vi "async worker process.vi"(10 "run flag in":u8 format="%.0b", 11 "module data in":T1={"run state"=enum."sync", "module"=refnum, "module ref"=refnum, "async exec ref"={"command fifo"=refnum, "error fifo"=refnum, "input buffer"=refnum, "output buffer"=refnum, "process buffer"=refnum, "original dvrs"=[]}, "configuration ref"=refnum, "error"={"status"=FALSE, "code"=0, "source"=""}, "previous error code"=0, "input method"={"data table"={"Double"=[], "Single"=[], "I64"=[], "I32"=[], "I16"=[], "I8"=[], "U64"=[], "U32"=[], "U16"=[], "U8"=[], "Boolean"=[], "String"=[], "Array of Double"=[], "Array of Single"=[], "Array of I64"=[], "Array of I32"=[], "Array of I16"=[], "Array of I8"=[], "Array of U64"=[], "Array of U32"=[], "Array of U16"=[], "Array of U8"=[], "Array of Boolean"=[], "Array of String"=[]}, "transfer spec"=[]}, "output method"={"data table"={"Double"=[], "Single"=[], "I64"=[], "I32"=[], "I16"=[], "I8"=[], "U64"=[], "U32"=[], "U16"=[], "U8"=[], "Boolean"=[], "String"=[], "Array of Double"=[], "Array of Single"=[], "Array of I64"=[], "Array of I32"=[], "Array of I16"=[], "Array of I8"=[], "Array of U64"=[], "Array of U32"=[], "Array of U16"=[], "Array of U8"=[], "Array of Boolean"=[], "Array of String"=[]}, "transfer spec"=[]}, "process method parameters"={"data table"={"Double"=[], "Single"=[], "I64"=[], "I32"=[], "I16"=[], "I8"=[], "U64"=[], "U32"=[], "U16"=[], "U8"=[], "Boolean"=[], "String"=[], "Array of Double"=[], "Array of Single"=[], "Array of I64"=[], "Array of I32"=[], "Array of I16"=[], "Array of I8"=[], "Array of U64"=[], "Array of U32"=[], "Array of U16"=[], "Array of U8"=[], "Array of Boolean"=[], "Array of String"=[]}, "transfer spec"=[]}, "process method results"={"data table"={"Double"=[], "Single"=[], "I64"=[], "I32"=[], "I16"=[], "I8"=[], "U64"=[], "U32"=[], "U16"=[], "U8"=[], "Boolean"=[], "String"=[], "Array of Double"=[], "Array of Single"=[], "Array of I64"=[], "Array of I32"=[], "Array of I16"=[], "Array of I8"=[], "Array of U64"=[], "Array of U32"=[], "Array of U16"=[], "Array of U8"=[], "Array of Boolean"=[], "Array of String"=[]}, "transfer spec"=[]}, "fault handling"={"unknown"=[], "trivial"=[], "critical"=[], "recoverable"=[]}, "error report index "=-1}) -> (0 "error out":errorcluster, 2 "run flag out":u8 format="%.0b", 3 "module data out":T1={"run state"=enum."sync", "module"=refnum, "module ref"=refnum, "async exec ref"={"command fifo"=refnum, "error fifo"=refnum, "input buffer"=refnum, "output buffer"=refnum, "process buffer"=refnum, "original dvrs"=[]}, "configuration ref"=refnum, "error"={"status"=FALSE, "code"=0, "source"=""}, "previous error code"=0, "input method"={"data table"={"Double"=[], "Single"=[], "I64"=[], "I32"=[], "I16"=[], "I8"=[], "U64"=[], "U32"=[], "U16"=[], "U8"=[], "Boolean"=[], "String"=[], "Array of Double"=[], "Array of Single"=[], "Array of I64"=[], "Array of I32"=[], "Array of I16"=[], "Array of I8"=[], "Array of U64"=[], "Array of U32"=[], "Array of U16"=[], "Array of U8"=[], "Array of Boolean"=[], "Array of String"=[]}, "transfer spec"=[]}, "output method"={"data table"={"Double"=[], "Single"=[], "I64"=[], "I32"=[], "I16"=[], "I8"=[], "U64"=[], "U32"=[], "U16"=[], "U8"=[], "Boolean"=[], "String"=[], "Array of Double"=[], "Array of Single"=[], "Array of I64"=[], "Array of I32"=[], "Array of I16"=[], "Array of I8"=[], "Array of U64"=[], "Array of U32"=[], "Array of U16"=[], "Array of U8"=[], "Array of Boolean"=[], "Array of String"=[]}, "transfer spec"=[]}, "process method parameters"={"data table"={"Double"=[], "Single"=[], "I64"=[], "I32"=[], "I16"=[], "I8"=[], "U64"=[], "U32"=[], "U16"=[], "U8"=[], "Boolean"=[], "String"=[], "Array of Double"=[], "Array of Single"=[], "Array of I64"=[], "Array of I32"=[], "Array of I16"=[], "Array of I8"=[], "Array of U64"=[], "Array of U32"=[], "Array of U16"=[], "Array of U8"=[], "Array of Boolean"=[], "Array of String"=[]}, "transfer spec"=[]}, "process method results"={"data table"={"Double"=[], "Single"=[], "I64"=[], "I32"=[], "I16"=[], "I8"=[], "U64"=[], "U32"=[], "U16"=[], "U8"=[], "Boolean"=[], "String"=[], "Array of Double"=[], "Array of Single"=[], "Array of I64"=[], "Array of I32"=[], "Array of I16"=[], "Array of I8"=[], "Array of U64"=[], "Array of U32"=[], "Array of U16"=[], "Array of U8"=[], "Array of Boolean"=[], "Array of String"=[]}, "transfer spec"=[]}, "fault handling"={"unknown"=[], "trivial"=[], "critical"=[], "recoverable"=[]}, "error report index "=-1})   [LabVIEW 2013, in "main engine.lvlib"]
doc: "This VI is like a mini data engine for a single TBM. It communicates with the engine that spawned it using a RT FIFO containing a command with DVRs used for data exchange. The command determines what method to run and gets commanded by the engine.\n\nThe engine is therefore still responsible for scheduling the execution of each module, but the engine won't block for data to be returned. An Asynch module can run as fast as an engine, or as slow as is needed to perform the required functionality."
uses:
  main engine/main engine.lvlib
  main engine/full module data.ctl
  <vilib>/NI/Tag Bus Module Framework/runtime/TBM module execution interface.lvclass
  main engine/module run state.ctl
  asynchronous executor reference.ctl
  async message to executor.ctl
  Runtime/async command notification.ctl
  <vilib>/NI/Tag Bus/table/data table.ctl
  Runtime/async error info.ctl
  <vilib>/NI/Tag Bus Module Framework/runtime/error classification.ctl
  <vilib>/NI/Tag Bus Module Framework/module configuration/TBM module configuration.lvclass
  main engine/module method data.ctl
  <vilib>/NI/Tag Bus/table/transfer specification.ctl
  <vilib>/NI/Tag Bus/tag/Data Type.ctl
  main engine/fault handling spec.ctl
  Configuration/Error Actions.ctl
  <vilib>/NI/Tag Bus/table/data table.lvlib
  <vilib>/NI/Tag Bus/tag/tag descriptor.lvclass
  Configuration/Standard Engine Configuration.lvclass
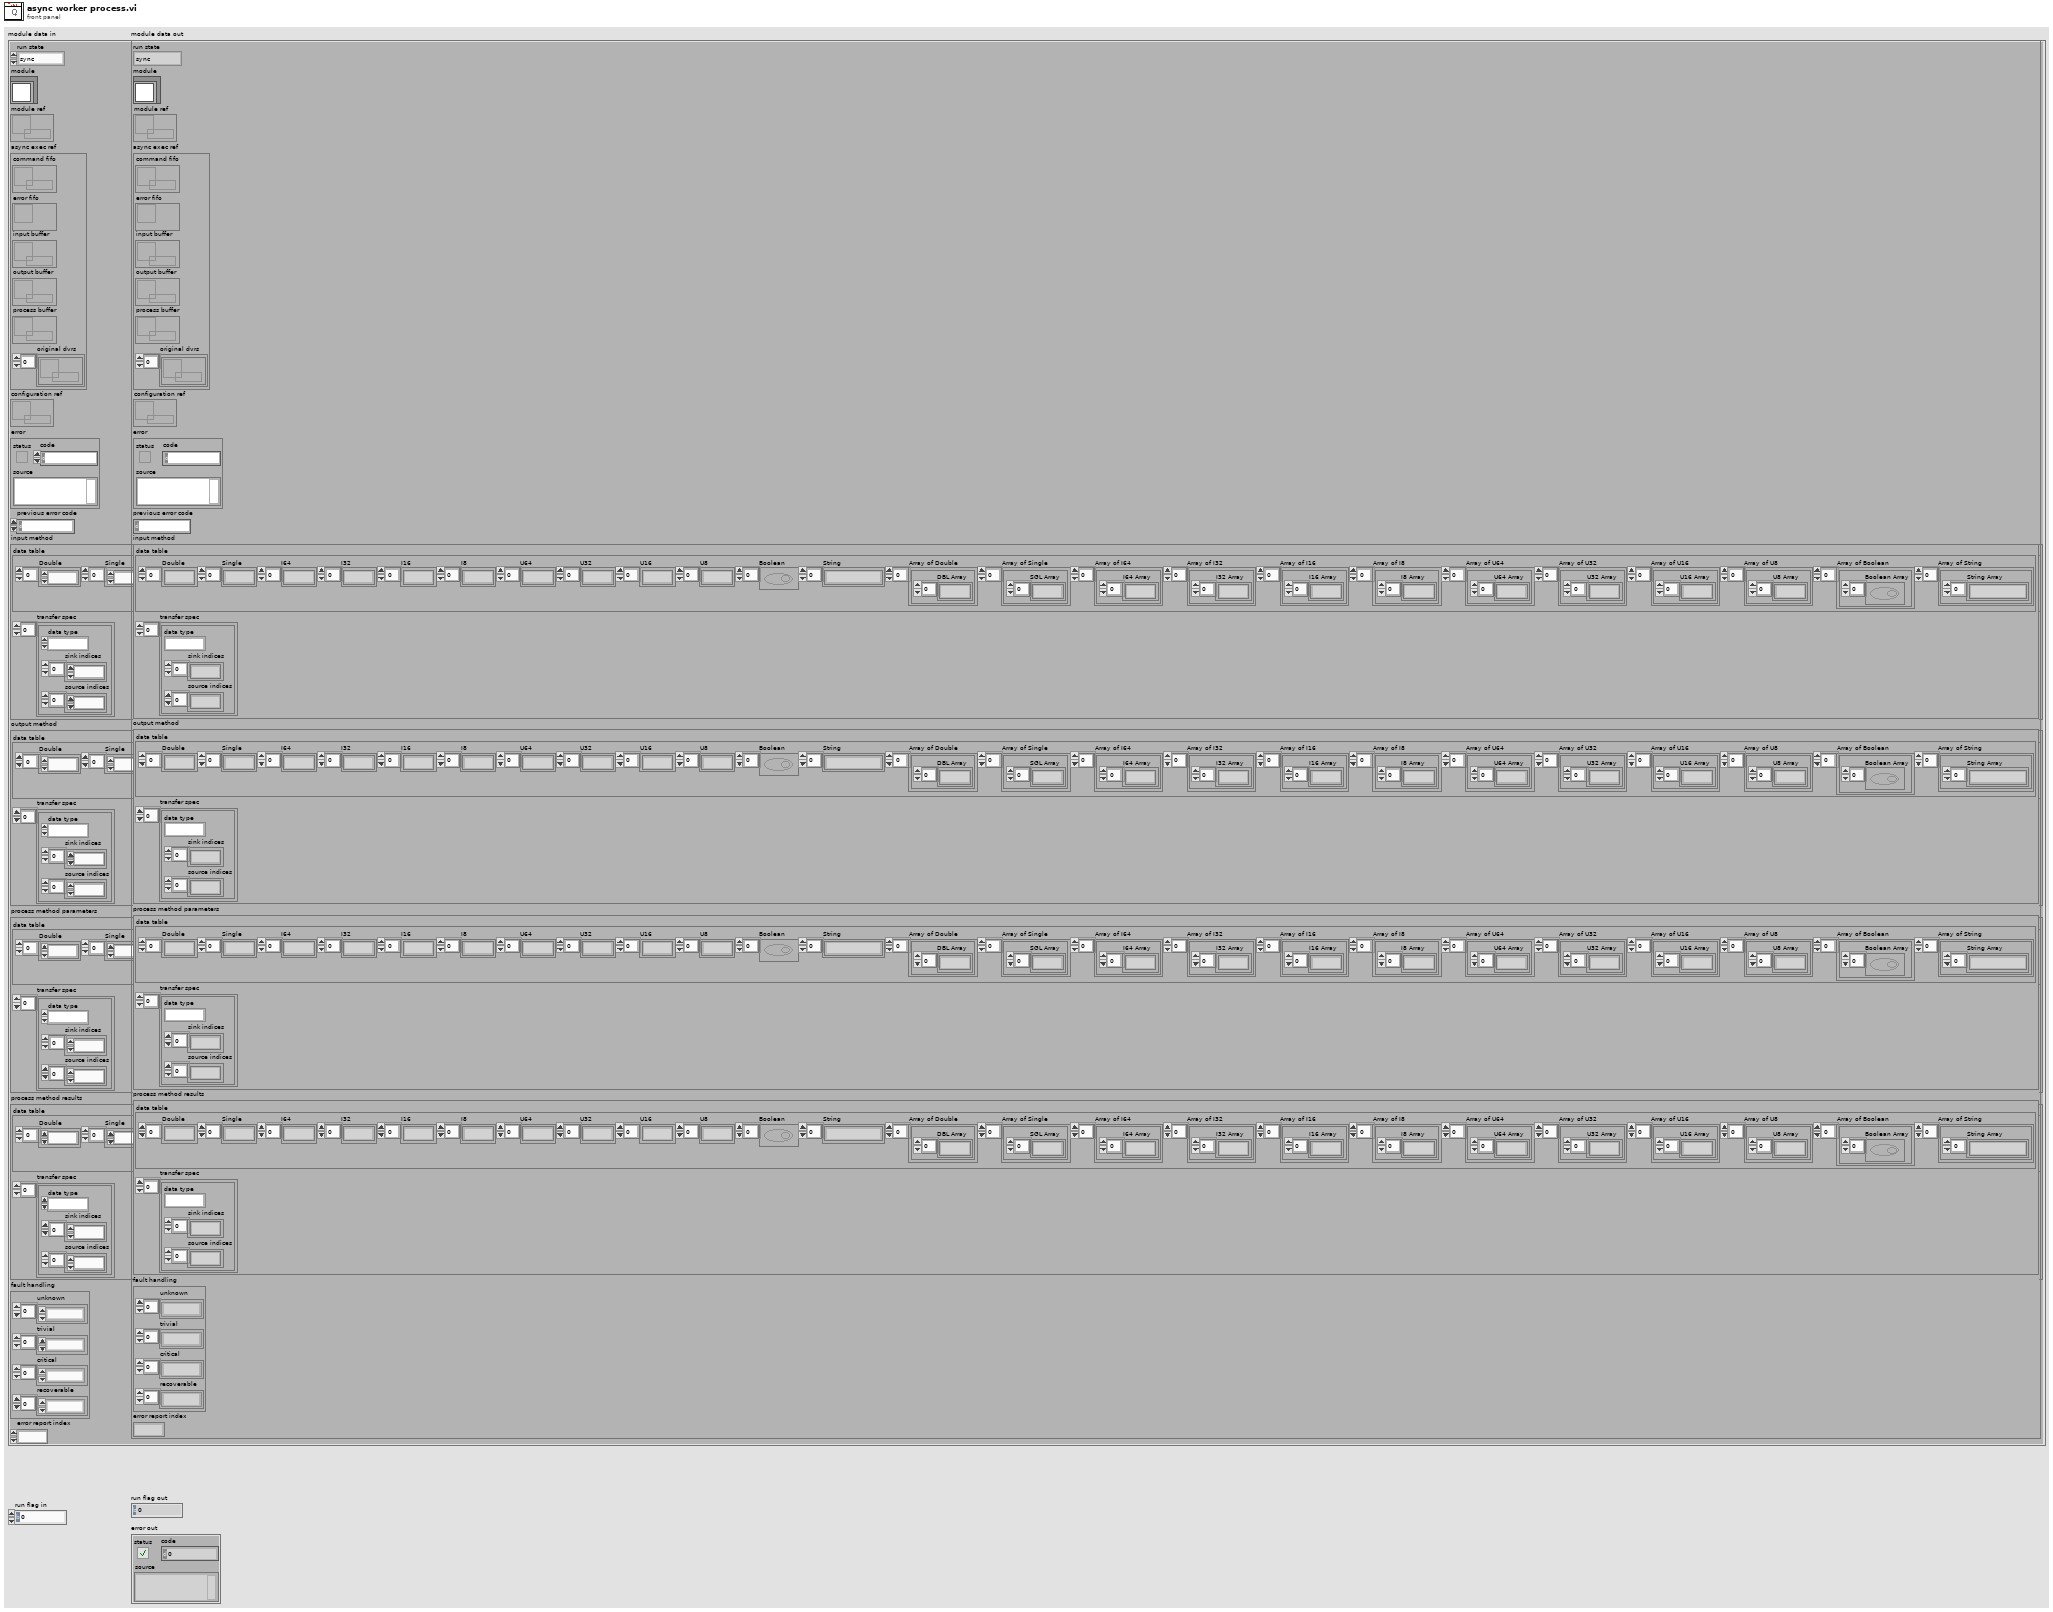
[diagram p1: front panel]
types:
  T1 = typedef "main engine.lvlib/full module data.ctl" = cluster{"run state":T2, "module":refnum<class "TBM module execution interface.lvclass">, "module ref":refnum<data-value>, "async exec ref":T3, "configuration ref":refnum<data-value>, "error":errorcluster, "previous error code":i32, "input method":T4, "output method":T4, "process method parameters":T4, "process method results":T4, "fault handling":T8, "error report index ":i32}
  T2 = typedef "main engine.lvlib/module run state.ctl" = enum16{"sync", "async"}
  T3 = typedef "main engine.lvlib/asynchronous executor reference.ctl" = cluster{"command fifo":refnum<k33>, "error fifo":refnum<k33>, "input buffer":refnum<k33>, "output buffer":refnum<k33>, "process buffer":refnum<k33>, "original dvrs":refnum<data-value>[]}
  T4 = typedef "main engine.lvlib/module method data.ctl" = cluster{"data table":T5, "transfer spec":T6[]}
  T5 = typedef "tag bus.lvlib/data table.lvlib/data table.ctl" = cluster{"Double":dbl[], "Single":sgl[], "I64":i64[], "I32":i32[], "I16":i16[], "I8":i8[], "U64":u64[], "U32":u32[], "U16":u16[], "U8":u8[], "Boolean":bool[], "String":string[], "Array of Double":cluster{"DBL Array":dbl[]}[], "Array of Single":cluster{"SGL Array":sgl[]}[], "Array of I64":cluster{"I64 Array":i64[]}[], "Array of I32":cluster{"I32 Array":i32[]}[], "Array of I16":cluster{"I16 Array":i16[]}[], "Array of I8":cluster{"I8 Array":i8[]}[], "Array of U64":cluster{"U64 Array":u64[]}[], "Array of U32":cluster{"U32 Array":u32[]}[], "Array of U16":cluster{"U16 Array":u16[]}[], "Array of U8":cluster{"U8 Array":u8[]}[], "Array of Boolean":cluster{"Boolean Array":bool[]}[], "Array of String":cluster{"String Array":string[]}[]}
  T6 = typedef "tag bus.lvlib/data table.lvlib/transfer specification.ctl" = cluster{"data type":T7, "sink indices":i32[], "source indices":i32[]}
  T7 = typedef "tag bus.lvlib/tag descriptor.lvclass/Data Type.ctl" = enum16{"Double", "Single", "I64", "I32", "I16", "I8", "U64", "U32", "U16", "U8", "Boolean", "String", "Array of Double", "Array of Single", "Array of I64", "Array of I32", "Array of I16", "Array of I8", "Array of U64", "Array of U32", "Array of U16", "Array of U8", "Array of Boolean", "Array of String"}
  T8 = typedef "main engine.lvlib/fault handling spec.ctl" = cluster{"unknown":T9[], "trivial":T9[], "critical":T9[], "recoverable":T9[]}
  T9 = typedef "Standard Engine Configuration.lvclass/Error Actions.ctl" = enum16{"Clear", "Notify", "Stop Component", "Stop Engine", "Safe State", "Attempt Recovery"}
  T10 = typedef "main engine.lvlib/async message to executor.ctl" = cluster{"command":T11, "data 1 (i,o,pp)":refnum<data-value>, "data 2 (pr)":refnum<data-value>, "user value":u64}
  T11 = typedef "main engine.lvlib/async command notification.ctl" = enum16{"stop", "input", "process", "output"}
  T12 = cluster{"parameters":refnum<data-value>, "results":refnum<data-value>}
  T13 = typedef "TBM module execution interface.lvclass/error classification.ctl" = enum16{"unknown", "none", "trivial", "recoverable", "critical"}
  T14 = typedef "main engine.lvlib/async error info.ctl" = cluster{"error code":i32, "error classification":T13}
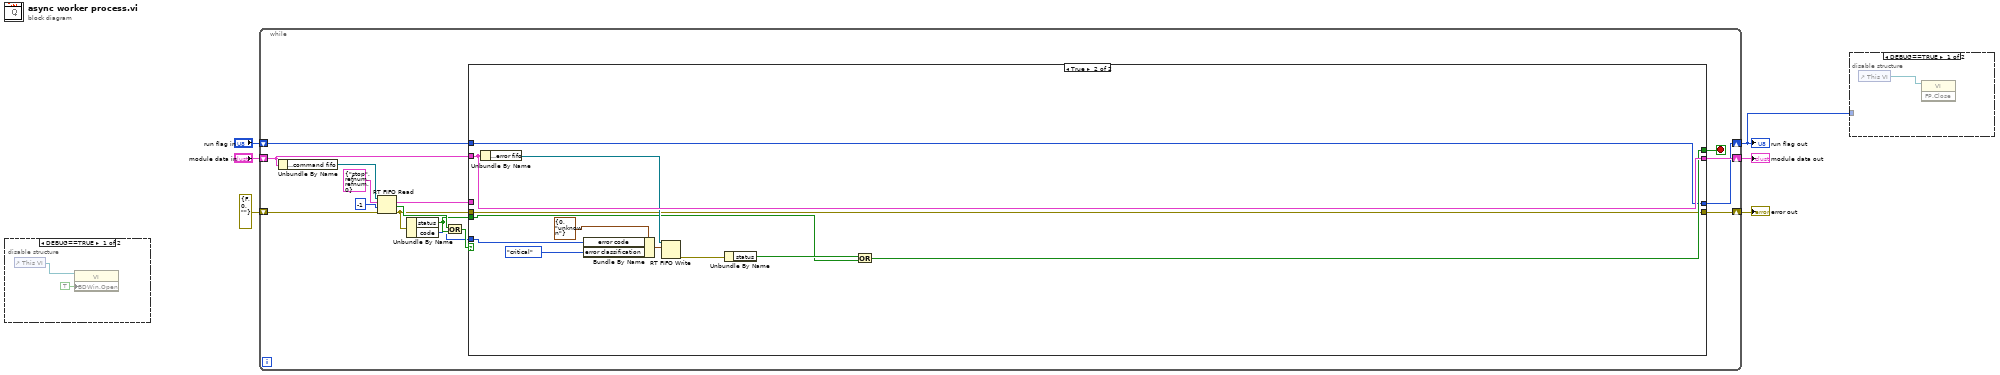
[diagram p0: block diagram]
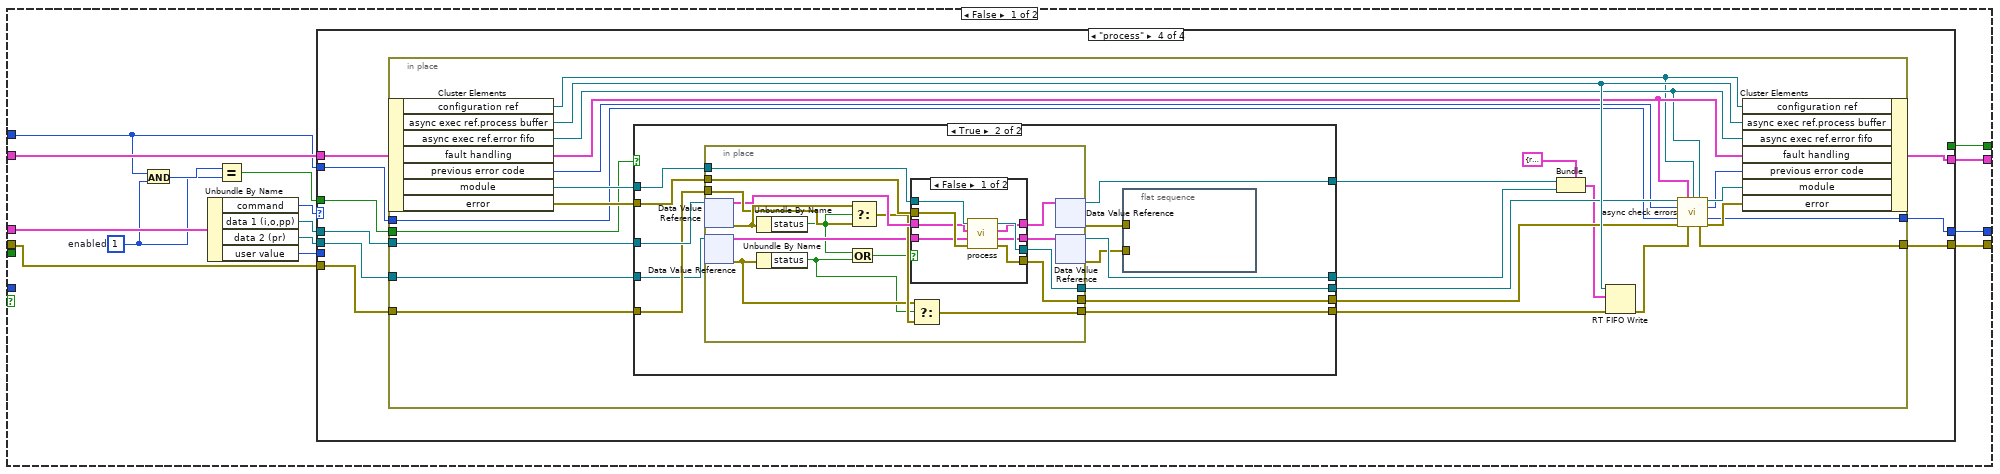
[diagram p4: hidden frame]
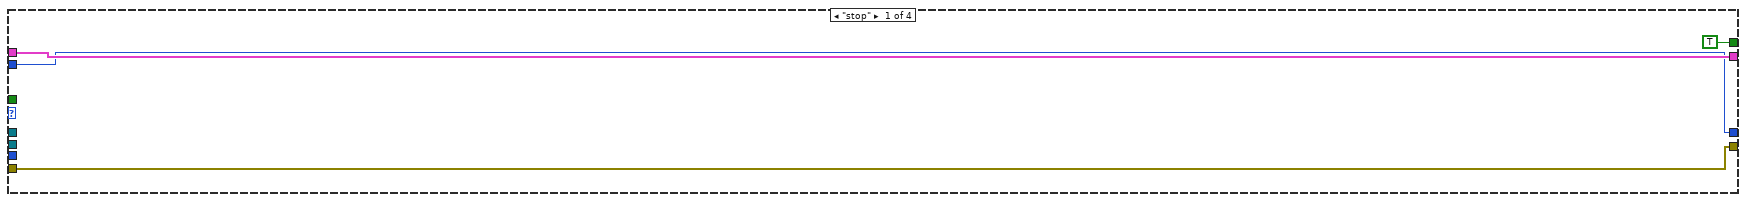
[diagram p5: hidden frame]
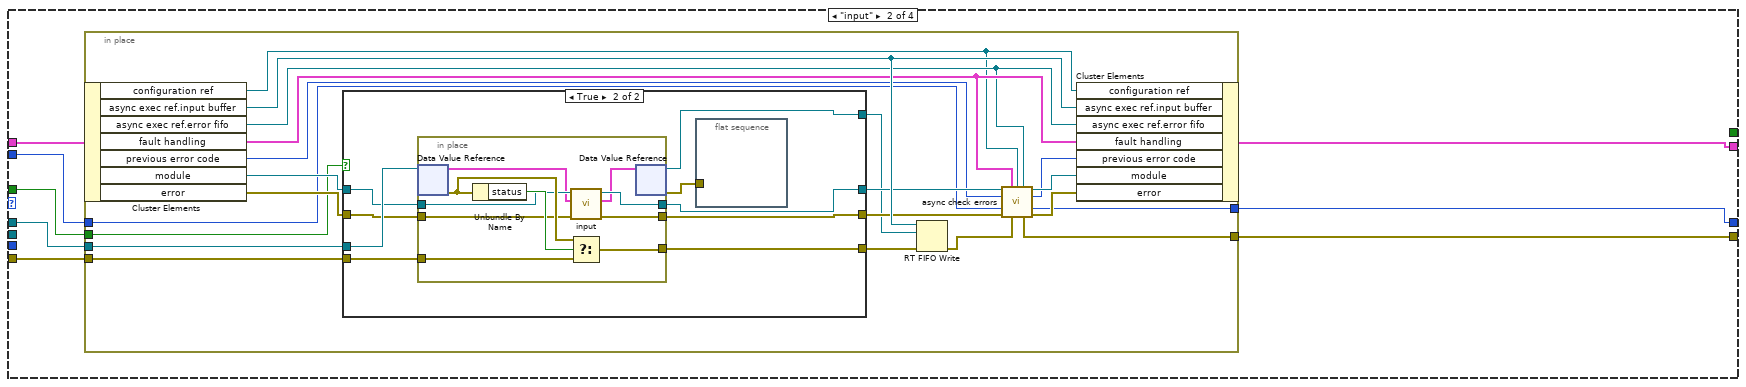
[diagram p6: hidden frame]
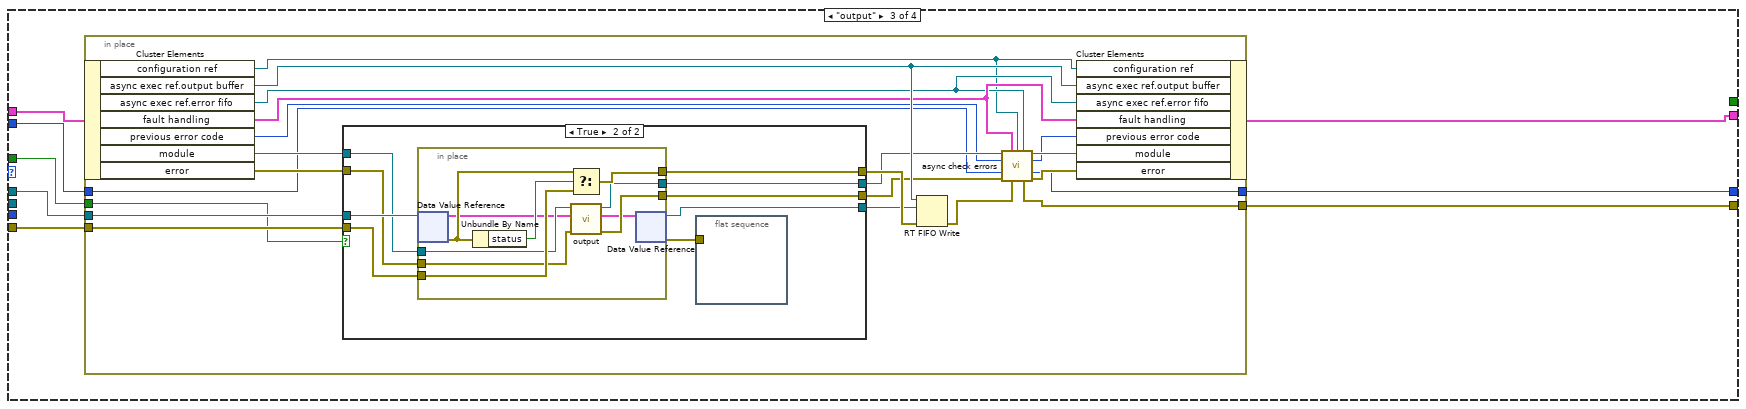
[diagram p8: hidden frame]
diagram:
  n1 = disable-structure shown="DEBUG==TRUE" {
    frame condition #0 {
      n2 = control-ref of="This VI"() -> (w8:refnum<vi>)
      n3 = property class="VI"(reference=w8, "BDWin.Open"=TRUE ("Block Diagram Window:Open")) -> ()  [unwired: 1 in, 2 out]
    }
    frame condition #1 (active) {
    }
  }
  n4 = while {
    shift-right: [w15] -> w5
    shift-left: "module data in" -> [w18]
    shift-right: [w12] -> w3
    shift-left: errorcluster {"status"=FALSE, "code"=0, "source"=""} ("error out") -> [w10]
    shift-right: [w9] -> w1
    shift-left: "run flag in" -> [w13]
    stop <- w14 stop-if-true
    n5 = Unbundle By Name(w18) -> ("async exec ref.command fifo"=w24:refnum<k33>)
    n6 = RT FIFO Read(0:w24, 1:T10 {"command"=enum."stop", "data 1 (i,o,pp)"=refnum, "data 2 (pr)"=refnum, "user value"=0} ("element"), 2:-1 ("timeout in ms (0)"), 3:w10) -> (9:w22:T10, 10:w20:bool, 11:w11:errorcluster)  [unwired: 2 out]
    n7 = Unbundle By Name(w11) -> ("status"=w17:bool, "code"=w16:i32)
    n8 = Or(x=w20, y=w17) -> (x .or. y?=w19:bool)
    n9 = case shown="True" w19 {
      tunnel: w22 -> [w39 _]
      tunnel: w18 -> [w37 w238]
      tunnel: w17 -> [_ w229]
      tunnel: w16 -> [_ w232]
      tunnel: [w36 w238] -> w15
      tunnel: [w35 w234] -> w14
      tunnel: [w32 w230] -> w9
      tunnel: w13 -> [w28 w230]
      tunnel: [w33 w228] -> w12
      tunnel: w11 -> [w34 w228]
      frame False {
        w26 = u8 1  # enabled
        n10 = And(x=w28, y=w26) -> (x .and. y?=w27:u8)
        n11 = Unbundle By Name(w39) -> ("command"=w38:T11, "data 1 (i,o,pp)"=w31:refnum<data-value>, "data 2 (pr)"=w30:refnum<data-value>, "user value"=w29:u64)
        n12 = Equal?(x=w27, y=w26) -> (x = y?=w25:bool)
        n13 = case shown="\"process\"" w38 {
          tunnel: w37 -> [w43 w51 w103 w156]
          tunnel: [w43 w50 w102 w155] -> w36
          tunnel: [TRUE _ _ _] -> w35
          tunnel: w34 -> [w41 w48 w100 w153]
          tunnel: [w41 w49 w101 w154] -> w33
          tunnel: [w40 w45 w97 w150] -> w32
          tunnel: w28 -> [w40 w46 w98 w151]
          tunnel: w31 -> [_ w47 w99 w152]
          tunnel: w30 -> [_ _ _ w149]
          tunnel: w29 -> [_ _ _ _]
          tunnel: w25 -> [_ w44 w96 w148]
          frame "stop" {
          }
          frame "input" {
            n14 = in-place {
              in-place-border: [w54] -> w49
              in-place-border: w48 -> [w70]
              in-place-border: w47 -> [w71]
              in-place-border: w46 -> [w60]
              in-place-border: [w59] -> w45
              in-place-border: w44 -> [w52]
              n15 = in-place-cluster #1(w51) -> ("configuration ref"=w53:refnum<data-value>, "async exec ref.input buffer"=w72:refnum<k33>, "async exec ref.error fifo"=w58:refnum<k33>, "fault handling"=w62:T8, "previous error code"=w57:i32, "module"=w68:refnum<class "TBM module execution interface.lvclass">, "error"=w67:errorcluster)
              n16 = case shown="True" w52 {
                tunnel: w71 -> [w73 w85]
                tunnel: w70 -> [w74 w84]
                tunnel: [w74 w83] -> w69
                tunnel: w68 -> [w76 w81]
                tunnel: w67 -> [w75 w80]
                tunnel: [w76 w79] -> w65
                tunnel: [w75 w78] -> w64
                tunnel: [w73 w77] -> w61
                frame False {
                }
                frame True {
                  n17 = in-place {
                    in-place-border: w84 -> [w93]
                    in-place-border: [w92] -> w83
                    in-place-border: [w91] -> w79
                    in-place-border: w81 -> [w90]
                    in-place-border: w80 -> [w89]
                    in-place-border: [w88] -> w78
                    n18 = in-place-dvr #2(w85) -> (w86:T5, w94:errorcluster)
                    n19 = Unbundle By Name(w94) -> ("status"=w95:bool)
                    n20 = call-dynamic "input.vi"("error in"=w89, "input allocation"=w86, "module in"=w90) -> ("error out"=w88:errorcluster, "input data"=w87:T5, "module out"=w91:refnum<class "TBM module execution interface.lvclass">)  [unwired: 6 in]
                    n21 = Select(t=w94, s=w95, f=w93) -> (s? t:f=w92:errorcluster)
                    n22 = in-place-dvr #2(w87) -> (w77:refnum<data-value>, w82:errorcluster)
                  }
                  n23 = flat-sequence {
                    tunnel: w82 -> [_]
                    frame #0 {
                    }
                  }
                }
              }
              n24 = RT FIFO Write(0:w72, 1:w61, 3:w69) -> (11:w55:errorcluster)  [unwired: 2 in, 3 out]
              n25 = call "async check errors.vi"("module in"=w65, "fault handling"=w62, "configuration ref"=w53, "error fifo"=w58, "previous error code in"=w57, "run flag in"=w60, "error in"=w64, "engine error in"=w55) -> ("module out"=w66:refnum<class "TBM module execution interface.lvclass">, "previous error code out"=w56:i32, "run flag out"=w59:u8, "engine error out"=w54:errorcluster, "error out"=w63:errorcluster)  [unwired: 3 in]
              n26 = in-place-cluster #1("configuration ref"=w53, "async exec ref.input buffer"=w72, "async exec ref.error fifo"=w58, "fault handling"=w62, "previous error code"=w56, "module"=w66, "error"=w63) -> (w50:T1)
            }
          }
          frame "output" {
            n27 = in-place {
              in-place-border: [w106] -> w101
              in-place-border: w100 -> [w122]
              in-place-border: w99 -> [w123]
              in-place-border: w98 -> [w112]
              in-place-border: [w111] -> w97
              in-place-border: w96 -> [w104]
              n28 = in-place-cluster #3(w103) -> ("configuration ref"=w105:refnum<data-value>, "async exec ref.output buffer"=w124:refnum<k33>, "async exec ref.error fifo"=w110:refnum<k33>, "fault handling"=w114:T8, "previous error code"=w109:i32, "module"=w120:refnum<class "TBM module execution interface.lvclass">, "error"=w119:errorcluster)
              n29 = case shown="True" w104 {
                tunnel: w123 -> [w125 w137]
                tunnel: w122 -> [w126 w136]
                tunnel: [w126 w135] -> w121
                tunnel: w120 -> [w128 w133]
                tunnel: w119 -> [w127 w132]
                tunnel: [w128 w131] -> w117
                tunnel: [w127 w130] -> w116
                tunnel: [w125 w129] -> w113
                frame False {
                }
                frame True {
                  n30 = in-place {
                    in-place-border: w136 -> [w145]
                    in-place-border: [w144] -> w135
                    in-place-border: [w143] -> w131
                    in-place-border: w133 -> [w142]
                    in-place-border: w132 -> [w141]
                    in-place-border: [w140] -> w130
                    n31 = in-place-dvr #4(w137) -> (w138:T5, w146:errorcluster)
                    n32 = Unbundle By Name(w146) -> ("status"=w147:bool)
                    n33 = Select(t=w146, s=w147, f=w145) -> (s? t:f=w144:errorcluster)
                    n34 = call-dynamic "output.vi"("error in"=w141, "output data"=w138, "module in"=w142) -> ("error out"=w140:errorcluster, "output allocation"=w139:T5, "module out"=w143:refnum<class "TBM module execution interface.lvclass">)  [unwired: 6 in]
                    n35 = in-place-dvr #4(w139) -> (w129:refnum<data-value>, w134:errorcluster)
                  }
                  n36 = flat-sequence {
                    tunnel: w134 -> [_]
                    frame #0 {
                    }
                  }
                }
              }
              n37 = RT FIFO Write(0:w124, 1:w113, 3:w121) -> (11:w107:errorcluster)  [unwired: 2 in, 3 out]
              n38 = call "async check errors.vi"("module in"=w117, "fault handling"=w114, "configuration ref"=w105, "error fifo"=w110, "previous error code in"=w109, "run flag in"=w112, "error in"=w116, "engine error in"=w107) -> ("module out"=w118:refnum<class "TBM module execution interface.lvclass">, "previous error code out"=w108:i32, "run flag out"=w111:u8, "engine error out"=w106:errorcluster, "error out"=w115:errorcluster)  [unwired: 3 in]
              n39 = in-place-cluster #3("configuration ref"=w105, "async exec ref.output buffer"=w124, "async exec ref.error fifo"=w110, "fault handling"=w114, "previous error code"=w108, "module"=w118, "error"=w115) -> (w102:T1)
            }
          }
          frame "process" {
            n40 = in-place {
              in-place-border: [w159] -> w154
              in-place-border: w153 -> [w179]
              in-place-border: w152 -> [w180]
              in-place-border: w151 -> [w170]
              in-place-border: [w169] -> w150
              in-place-border: w149 -> [w168]
              in-place-border: w148 -> [w157]
              n41 = in-place-cluster #5(w156) -> ("configuration ref"=w158:refnum<data-value>, "async exec ref.process buffer"=w181:refnum<k33>, "async exec ref.error fifo"=w163:refnum<k33>, "fault handling"=w171:T8, "previous error code"=w162:i32, "module"=w177:refnum<class "TBM module execution interface.lvclass">, "error"=w176:errorcluster)
              n42 = case shown="True" w157 {
                tunnel: w180 -> [w183 w198]
                tunnel: w179 -> [w184 w197]
                tunnel: [w184 w196] -> w178
                tunnel: w177 -> [w186 w194]
                tunnel: w176 -> [w185 w193]
                tunnel: [w186 w192] -> w174
                tunnel: [w185 w191] -> w173
                tunnel: w168 -> [w182 w190]
                tunnel: [w183 w189] -> w165
                tunnel: [w182 w188] -> w164
                frame False {
                }
                frame True {
                  n43 = in-place {
                    in-place-border: w197 -> [w213]
                    in-place-border: [w205] -> w196
                    in-place-border: [w212] -> w192
                    in-place-border: w194 -> [w211]
                    in-place-border: w193 -> [w210]
                    in-place-border: [w209] -> w191
                    n44 = in-place-dvr #6(w198) -> (w207:T5, w214:errorcluster)
                    n45 = in-place-dvr #7(w190) -> (w203:T5, w204:errorcluster)
                    n46 = Unbundle By Name(w214) -> ("status"=w201:bool)
                    n47 = Unbundle By Name(w204) -> ("status"=w200:bool)
                    n48 = Or(x=w201, y=w200) -> (x .or. y?=w199:bool)
                    n49 = Select(t=w214, s=w201, f=w213) -> (s? t:f=w206:errorcluster)
                    n50 = case shown="False" w199 {
                      tunnel: [w222 w226] -> w212
                      tunnel: w211 -> [w221 w226]
                      tunnel: w210 -> [w220 w225]
                      tunnel: [w219 w225] -> w209
                      tunnel: [w218 w223] -> w208
                      tunnel: w207 -> [w217 w223]
                      tunnel: w203 -> [w216 w224]
                      tunnel: [w215 w224] -> w202
                      frame False {
                        n51 = call-dynamic "process.vi"("error in"=w220, "result allocation"=w216, "parameters"=w217, "module in"=w221) -> ("error out"=w219:errorcluster, "results"=w215:T5, "parameter allocation"=w218:T5, "module out"=w222:refnum<class "TBM module execution interface.lvclass">)  [unwired: 4 in]
                      }
                      frame True {
                      }
                    }
                    n52 = Select(t=w204, s=w200, f=w206) -> (s? t:f=w205:errorcluster)
                    n53 = in-place-dvr #6(w208) -> (w189:refnum<data-value>, w195:errorcluster)
                    n54 = in-place-dvr #7(w202) -> (w188:refnum<data-value>, w187:errorcluster)
                  }
                  n55 = flat-sequence {
                    tunnel: w195 -> [_]
                    tunnel: w187 -> [_]
                    frame #0 {
                    }
                  }
                }
              }
              n56 = Bundle(cluster=T12 {"parameters"=refnum, "results"=refnum} ("element"), "parameters"=w165, "results"=w164) -> (w166:T12)
              n57 = RT FIFO Write(0:w181, 1:w166, 3:w178) -> (11:w160:errorcluster)  [unwired: 2 in, 3 out]
              n58 = call "async check errors.vi"("module in"=w174, "fault handling"=w171, "configuration ref"=w158, "error fifo"=w163, "previous error code in"=w162, "run flag in"=w170, "error in"=w173, "engine error in"=w160) -> ("module out"=w175:refnum<class "TBM module execution interface.lvclass">, "previous error code out"=w161:i32, "run flag out"=w169:u8, "engine error out"=w159:errorcluster, "error out"=w172:errorcluster)  [unwired: 3 in]
              n59 = in-place-cluster #5("configuration ref"=w158, "async exec ref.process buffer"=w181, "async exec ref.error fifo"=w163, "fault handling"=w171, "previous error code"=w161, "module"=w175, "error"=w172) -> (w155:T1)
            }
          }
        }
      }
      frame True {
        n60 = Unbundle By Name(w238) -> ("async exec ref.error fifo"=w237:refnum<k33>)
        n61 = Bundle By Name(cluster=T14 {"error code"=0, "error classification"=enum."unknown"} ("element"), "error code"=w232, "error classification"=error_classification."critical") -> (w233:T14)
        n62 = RT FIFO Write(0:w237, 1:w233) -> (11:w227:errorcluster)  [unwired: 3 in, 3 out]
        n63 = Unbundle By Name(w227) -> ("status"=w235:bool)
        n64 = Or(x=w235, y=w229) -> (x .or. y?=w234:bool)
      }
    }
  }
  "module data out" <- w5
  "error out" <- w3
  "run flag out" <- w1
  n65 = disable-structure shown="DEBUG==TRUE" {
    disable-tunnel: w1 -> [_ _]
    frame condition #0 {
      n66 = control-ref of="This VI"() -> (w239:refnum<vi>)
      n67 = invoke class="VI" method="FP.Close"(reference=w239) -> ()  [unwired: 2 in, 3 out]
    }
    frame condition #1 (active) {
    }
  }
